vi "Read RC parameters_default_UI.vi"(0 "JSON FilePath":path=path "F:/User Interface Testbench/Configuration file/Rack Controller Override JSON UI.json", 1 "ListBox Cluster":T1, 5 "Rack Id":string="0", 7 "Variant":variant, 9 "Part Name":string, 11 "error in (no error)":errorcluster, 12 "Variant?":bool) -> (4 "Output Edit Tolerance cluster":T1, 6 "Error Message":string, 15 "error out":errorcluster)   [LabVIEW 2019, in "ZenGage v3.0 UI.lvclass"]
uses:
  ZenGage v3.0 UI.lvclass
  Type Definitions/Edit tolerance settings/Rack Selection.ctl
  <vilib>/Utility/miscctls.llb/LVPoint32TypeDef.ctl
  Type Definitions/Edit tolerance settings/Edit Tolerance Input.ctl
panel:
  out "VCluster\n out":variant
  # "e"
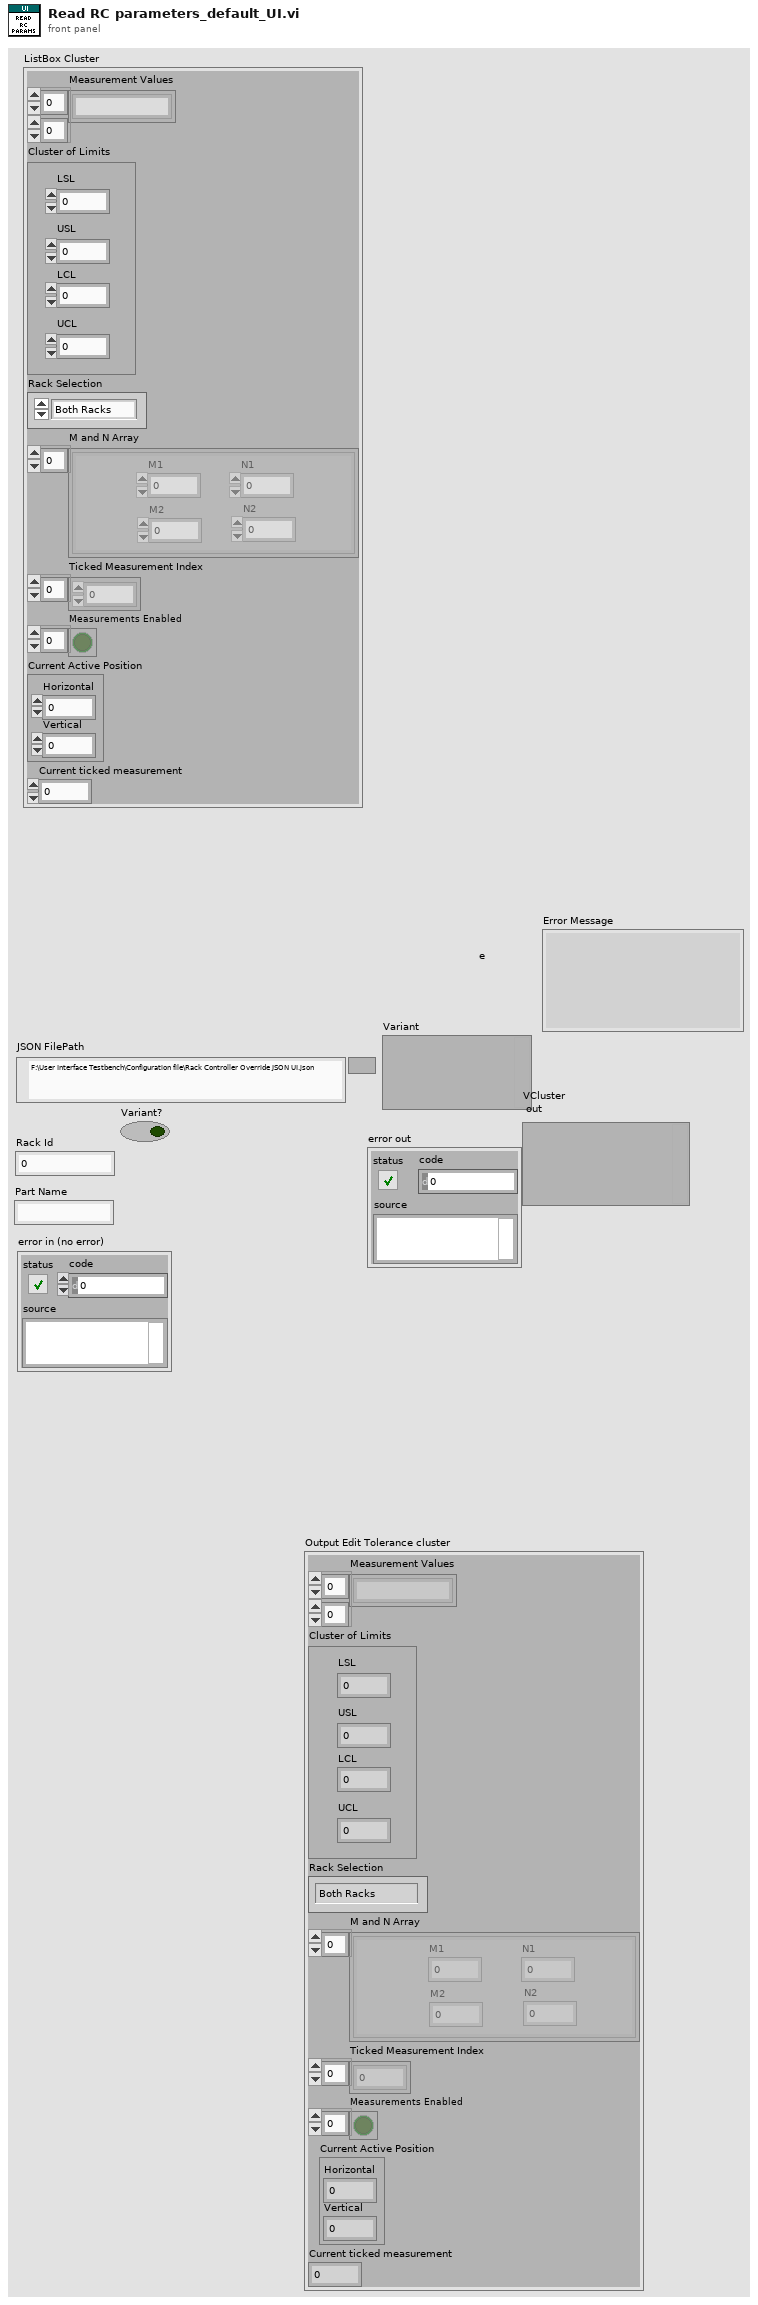
[diagram p1: front panel]
types:
  T1 = typedef "ZenGage v3.0 UI.lvclass/Edit Tolerance Input.ctl" = cluster{"Measurement Values":string[][], "Cluster of Limits":cluster{"LSL":dbl, "USL":dbl, "LCL":dbl, "UCL":dbl}, "Rack Selection":T2, "M and N Array":cluster{"M1":u64, "M2":u64, "N1":u64, "N2":u64}[], "Ticked Measurement Index":u32[], "Measurements Enabled":bool[], "Current Active Position":T3, "Current ticked measurement":dbl}
  T2 = typedef "ZenGage v3.0 UI.lvclass/Rack Selection.ctl" = enum16{"Both Racks", "Rack 2", "Rack 1"}
  T3 = typedef "LVPoint32TypeDef.ctl" = cluster{"Horizontal":i32, "Vertical":i32}
  T4 = cluster{"Name":string, "Measurements":cluster{"MeasurementId":dbl, "Name":string, "ControlLimitsViolationThreshold":cluster{"AllowableFails":dbl, "WindowSize":dbl}, "SpecificationLimitViolationThreshold":cluster{"AllowableFails":dbl, "WindowSize":dbl}}[], "UnloadPositionCounts":cluster{"Fail":dbl, "ReelEnd":dbl, "ProductionEnd":dbl}}
  T5 = cluster{cluster{"Name":string, "Measurements":cluster{"MeasurementId":dbl, "Name":string, "ControlLimitsViolationThreshold":cluster{"AllowableFails":dbl, "WindowSize":dbl}, "SpecificationLimitViolationThreshold":cluster{"AllowableFails":dbl, "WindowSize":dbl}}[], "UnloadPositionCounts":cluster{"Fail":dbl, "ReelEnd":dbl, "ProductionEnd":dbl}}}
  T6 = cluster{"MeasurementId":dbl, "Name":string, "ControlLimitsViolationThreshold":cluster{"AllowableFails":dbl, "WindowSize":dbl}, "SpecificationLimitViolationThreshold":cluster{"AllowableFails":dbl, "WindowSize":dbl}}[]
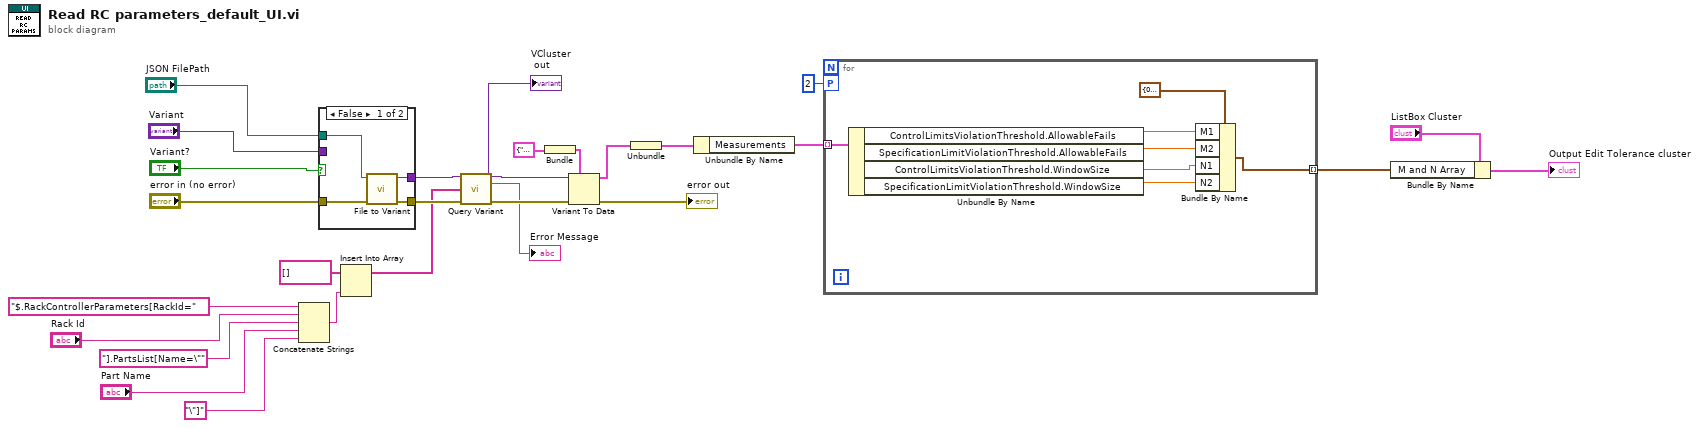
[diagram p0: block diagram]
diagram:
  n1 = Concatenate Strings("$.RackControllerParameters[RackId=" ("string"), "Rack Id", "].PartsList[Name=\"" ("string"), "Part Name", "\"]" ("string")) -> (w14:string)
  n2 = case shown="False" "Variant?" {
    tunnel: [w31 w33] -> w27
    tunnel: "error in (no error)" -> [w30 w33]
    tunnel: [w29 w32] -> w22
    tunnel: "JSON FilePath" -> [w28 _]
    tunnel: "Variant" -> [_ w32]
    frame False {
      n3 = call <vilib>:"File to Variant.vi"("JSON FilePath"=w28, "error in (no error)"=w30) -> ("JSON Variant"=w29:variant, "error out"=w31:errorcluster)  [unwired: 6 in, 1 out]
    }
    frame True {
    }
  }
  n4 = Insert Into Array(array=string[] [], new element=w14) -> (w12:string[])  [unwired: 1 in]
  n5 = call <vilib>:"Query Variant.vi"("VCluster in"=w22, "pathList"=w12, "error IO"=w27) -> ("VCluster\n out"=w23:variant, "Error Message"=→"Error Message":string, "error out"=w25:errorcluster)  [unwired: 9 in, 1 out]
  "VCluster\n out" <- w23
  n6 = Bundle(T4 {"Name"="", "Measurements"=[], "UnloadPositionCounts"={"Fail"=0.0, "ReelEnd"=0.0, "ProductionEnd"=0.0}}) -> (w4:T5)  [unwired: 1 in]
  n7 = Variant To Data(error in=w25, type=w4, Variant=w23) -> (data=w3:T5, error out=→"error out":errorcluster)
  n8 = Unbundle(w3) -> (w2:T4)
  n9 = Unbundle By Name(w2) -> ("Measurements"=w10:T6)
  n10 = for {
    tunnel: w10 -> [w40] mode=indexing
    tunnel: [w34] -> w9 mode=indexing
    workers-P: 2 -> [_]
    n11 = Unbundle By Name(w40) -> ("ControlLimitsViolationThreshold.AllowableFails"=w38:dbl, "SpecificationLimitViolationThreshold.AllowableFails"=w37:dbl, "ControlLimitsViolationThreshold.WindowSize"=w36:dbl, "SpecificationLimitViolationThreshold.WindowSize"=w35:dbl)
    n12 = Bundle By Name(cluster=cluster{"M1":u64, "M2":u64, "N1":u64, "N2":u64} {"M1"=0, "M2"=0, "N1"=0, "N2"=0} ("Rack 1"), "M1"=w38, "M2"=w37, "N1"=w36, "N2"=w35) -> (w34:cluster{"M1":u64, "M2":u64, "N1":u64, "N2":u64})
  }
  n13 = Bundle By Name(cluster="ListBox Cluster", "M and N Array"=w9) -> (→"Output Edit Tolerance cluster":T1)
